vi "Test As RIO Server.vi"() -> ()   [LabVIEW 2019]
uses:
  <vilib>/FPGAPlugInAG/cRIO-9064/niLvFpga_Close_cRIO-9064.vi
  <vilib>/rvi/interface/nirviOpenFPGA/nirviOpenFPGA.xnode
  FPGA Bitfiles/examplefpgaproje_FPGATarget_FPGAMain_u8-CWS6Ina0.lvbitx
  <vilib>/rvi/interface/nirviReadWriteControl/nirviReadWriteControl.xnode
  <vilib>/rvi/interface/nirviCloseFPGA/nirviCloseFPGA.xnode
  <vilib>/FPGAPlugInAG/cRIO-9064/niLvFpga_Open_cRIO-9064.vi
  NiFpgaLv.dll
  <vilib>/Utility/error.llb/Error Cluster From Error Code.vi
  <vilib>/rvi/errors/niLvFpgaAdjustHostInterfaceError.vi
panel:
  out "error out":errorcluster
  out "U8 Result":u8
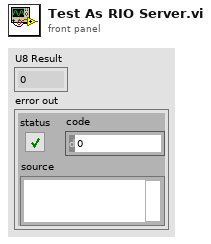
[diagram p1: front panel]
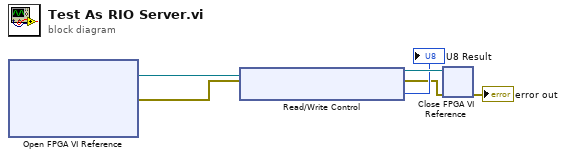
[diagram p0: block diagram]
diagram:
  n1 = xnode "Open FPGA VI Reference"() -> ("FPGA VI Reference Out"=w6:refnum<k20>, "error out"=w3:errorcluster)  [unwired: 2 in]
  n2 = xnode "Read/Write Control"("FPGA VI Reference In"=w6, "error in"=w3) -> ("FPGA VI Reference Out"=w5:refnum<k20>, "error out"=w2:errorcluster, "U8 Result"=→"U8 Result":u8)
  n3 = xnode "Close FPGA VI Reference"("FPGA VI Reference In"=w5, "error in"=w2) -> ("error out"=→"error out":errorcluster)
